vi "check network stream connection.vi"(11 "stream ref":refnum<k21>) -> (3 "Connected":bool)   [LabVIEW 2018]
uses:
  <resource>/objmgr/ni.dex.rc
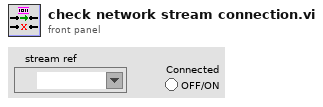
[diagram p1: front panel]
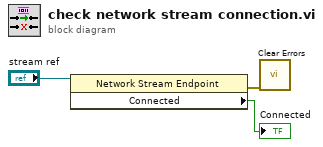
[diagram p0: block diagram]
diagram:
  n1 = property class="Network Stream Endpoint"(reference="stream ref") -> (error out=w3:errorcluster, "Connected"=→"Connected":bool)  [unwired: 1 in, 1 out]
  n2 = call <vilib>:"Clear Errors.vi"("error in (no error)"=w3) -> ()  [unwired: 5 in, 2 out]
